vi "LS330_QRY.vi"(8 "error in":errorcluster, 10 "CMD":string, 11 "VISA resource name":refnum<visa-resource-name>) -> (0 "error out":errorcluster, 1 "return count":u32, 2 "OUT":string, 3 "VISA resource name out":refnum<visa-resource-name>)   [LabVIEW 2021]
uses:
  31ca410e-eb9f-45fd-896e-dea07802b8d0.vi
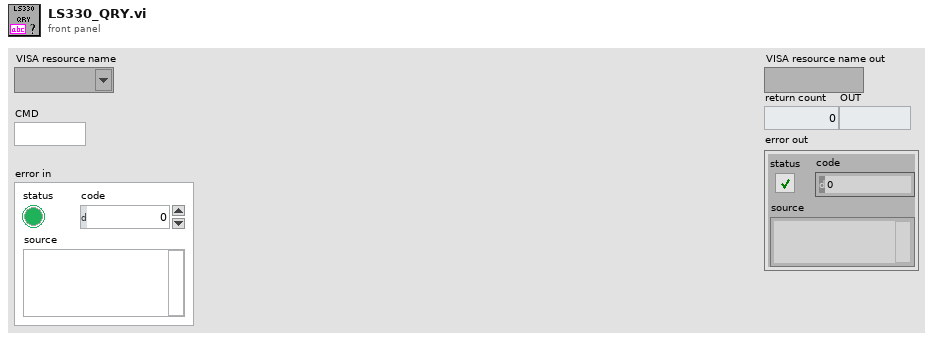
[diagram p1: front panel]
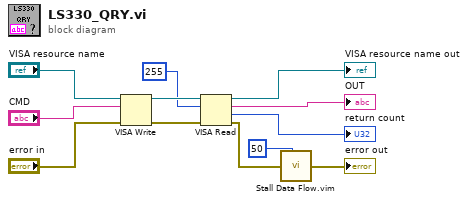
[diagram p0: block diagram]
diagram:
  n1 = VISA Write(VISA resource name="VISA resource name", write buffer="CMD", error in (no error)="error in") -> (VISA resource name out=w9:refnum<visa-resource-name>, error out=w8:errorcluster)  [unwired: 1 out]
  n2 = VISA Read(VISA resource name=w9, byte count=u32 255, error in (no error)=w8) -> (VISA resource name out=→"VISA resource name out":refnum<visa-resource-name>, read buffer=→"OUT":string, return count=→"return count":u32, error out=w6:errorcluster)
  n3 = call "Stall Data Flow.vim"("value in"=w6, "milliseconds to wait"=u32 50) -> ("value out"=→"error out":errorcluster)  [unwired: 1 out]
